vi "Read num2.vi"(8 "error in (no error)":errorcluster, 11 "AbsorbPOrigin in":refnum<class "AbsorbPOrigin.lvclass">) -> (0 "error out":errorcluster, 2 "num2":T1, 3 "AbsorbPOrigin out":refnum<class "AbsorbPOrigin.lvclass">)   [LabVIEW 2022 SP3, in "TCSDataDefinitions.lvlib" / "TCSCommand.lvlib" / "POriginCommands.lvlib" / "AbsorbPOrigin.lvclass"]
uses:
  AbsorbPOrigin.lvclass
  OffsetCommands/Enumerations/Num2Types.ctl
  AbsorbPOrigin.lvclass/AbsorbPOrigin.ctl
  OffsetCommands/OffsetCommands.lvlib
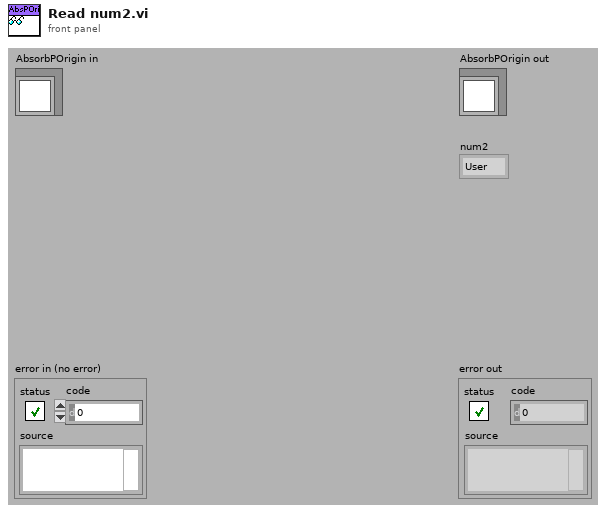
[diagram p1: front panel]
types:
  T1 = typedef "TCSDataDefinitions.lvlib/TCSCommand.lvlib/OffsetCommands.lvlib/Num2Types.ctl" = enum16{"User", "Handset", "Both"}
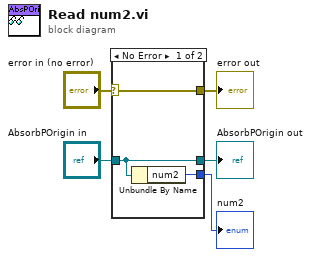
[diagram p0: block diagram]
diagram:
  n1 = case shown="No Error" "error in (no error)" {
    selector: "error in (no error)" -> [w8 w9]
    tunnel: [w8 w9] -> w4
    tunnel: [w7 w10] -> w2
    tunnel: "AbsorbPOrigin in" -> [w7 w10]
    tunnel: [w6 _] -> w1
    frame No Error {
      n2 = Unbundle By Name(w7) -> ("num2"=w6:T1)
    }
    frame Error {
    }
  }
  "error out" <- w4
  "AbsorbPOrigin out" <- w2
  "num2" <- w1
